vi "XY Graph Load Plot(s) Event.vi"(6 "Plot Format Information (dialog)":T1={"Number of Lines to Skip"=-1, "Column Header Line?"=FALSE, "Separator"="", "Abscissa Column?"=FALSE, "Abscissa Start"=nan, "Abscissa Step"=nan}, 7 "Max Number of Plot to Load (-1: All)":i32=-1, 8 "Error In":errorcluster, 9 "File Path":path, 10 "Used Dialog? (T)":bool=TRUE, 11 "XYGraph Ref":T2) -> (0 "Error Out":errorcluster, 1 "Message":string, 2 "File Path(s)":path[](array[path]), 3 "Loaded Plot Names":cluster{"Plot Names":string[]}[](array[cluster]), 4 "# Plots Added":i32[](array[numeric]), 5 "Graph Name":string)   [LabVIEW 2021, in "XY Graph Add-Ons.lvlib"]
uses:
  XY Graph Add-Ons.lvlib
  XY Graph Refnum.ctl
  XY Graph Plot Format Information.ctl
  Files/ASCII File Header Definition.ctl
  91129bd3-31c1-4cfb-ab33-95d83ad30e2f.vi
  0e8d2310-731b-4b54-9d07-3dcbb9077907.vi
  <vilib>/Utility/error.llb/Error Cluster From Error Code.vi
  XY Graph Get Plots Metadata.vi
  XY Graph Set Plots Metadata.vi
  <vilib>/ErrorRing/Error Ring.xnode
  Strings/Strings.lvlib
  Files/Files.lvlib
  Graphs.lvlib
  Error/Error.lvlib
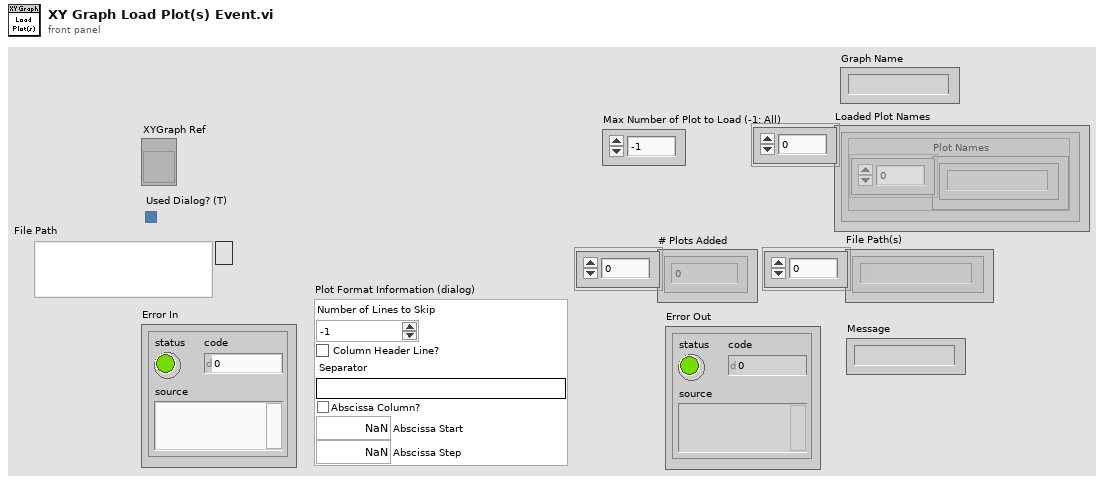
[diagram p1: front panel]
types:
  T1 = typedef "XY Graph Add-Ons.lvlib/XY Graph Plot Format Information.ctl" = cluster{"Number of Lines to Skip":i32, "Column Header Line?":bool, "Separator":string, "Abscissa Column?":bool, "Abscissa Start":dbl, "Abscissa Step":dbl}
  T2 = typedef "XY Graph Add-Ons.lvlib/XY Graph Refnum.ctl" = refnum<vi>
  T3 = typedef "Files.lvlib/ASCII File Header Definition.ctl" = cluster{"Number of Lines to Skip":i32, "Column Header Line?":bool}
  T4 = typedef "XY Graph Add-Ons.lvlib/XY Graph Plot Scale Labels.ctl" = cluster{"X Scale Label":string, "Y Scale Label":string}
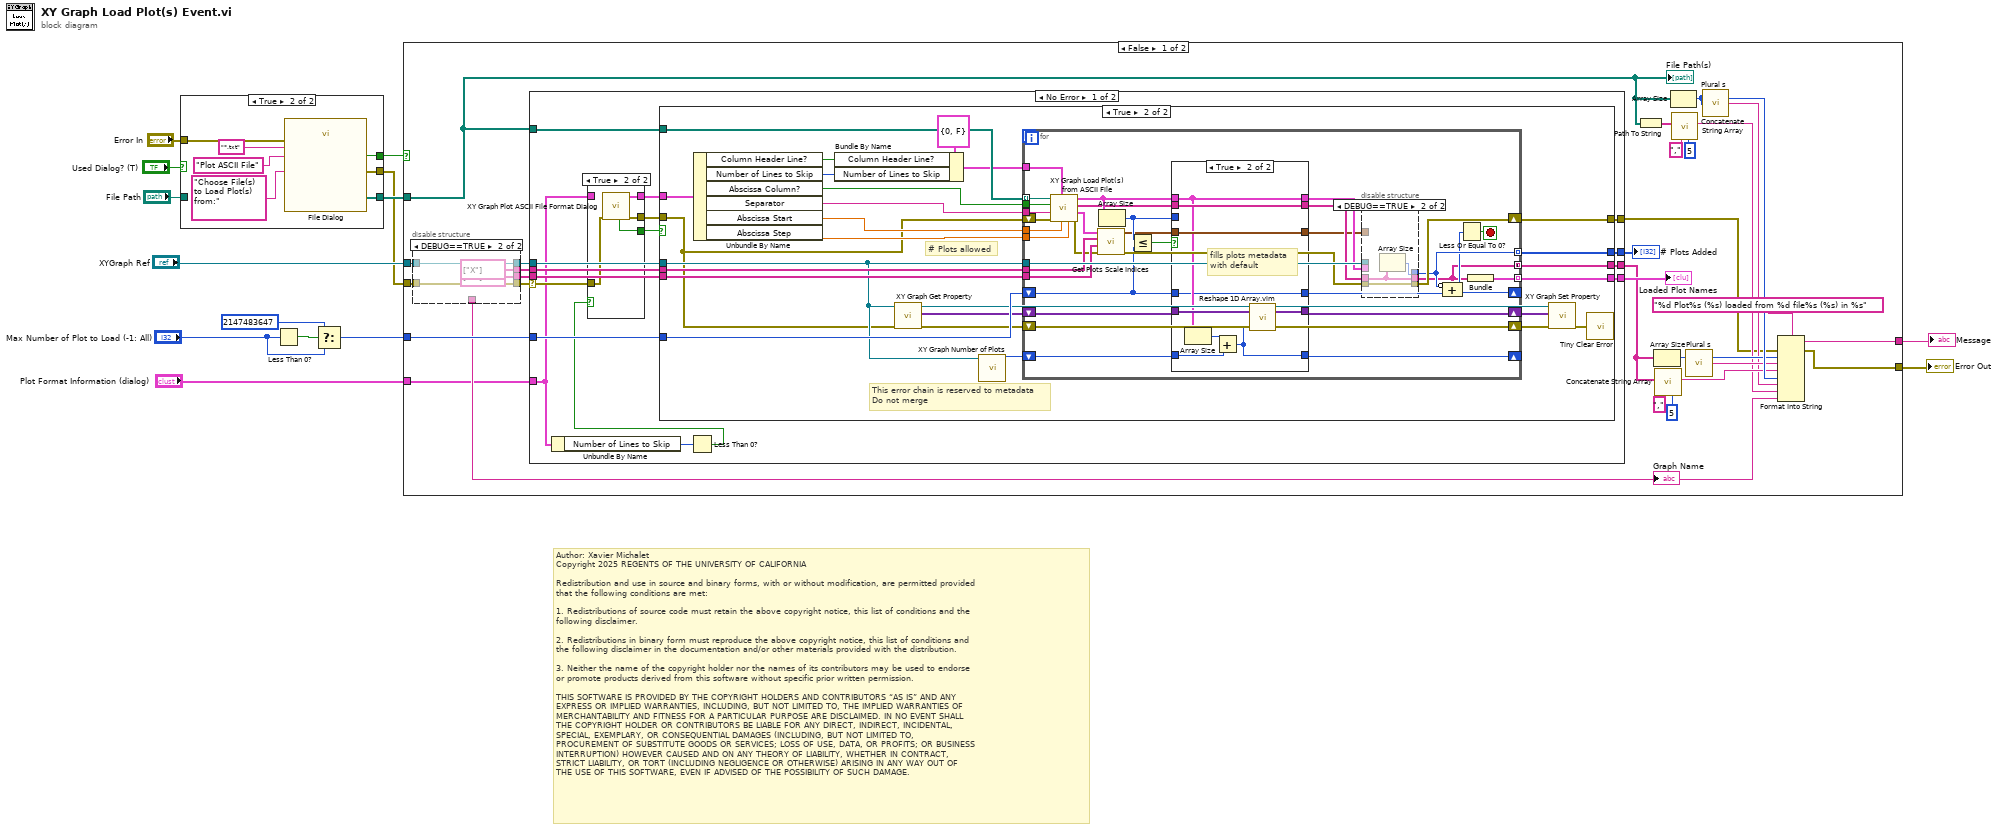
[diagram p0: block diagram]
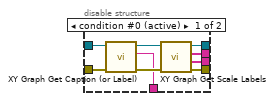
[diagram p2: hidden frame]
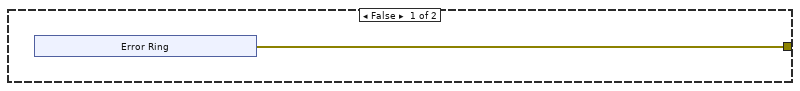
[diagram p4: hidden frame]
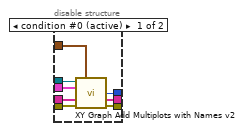
[diagram p5: hidden frame]
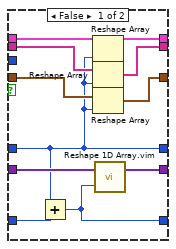
[diagram p6: hidden frame]
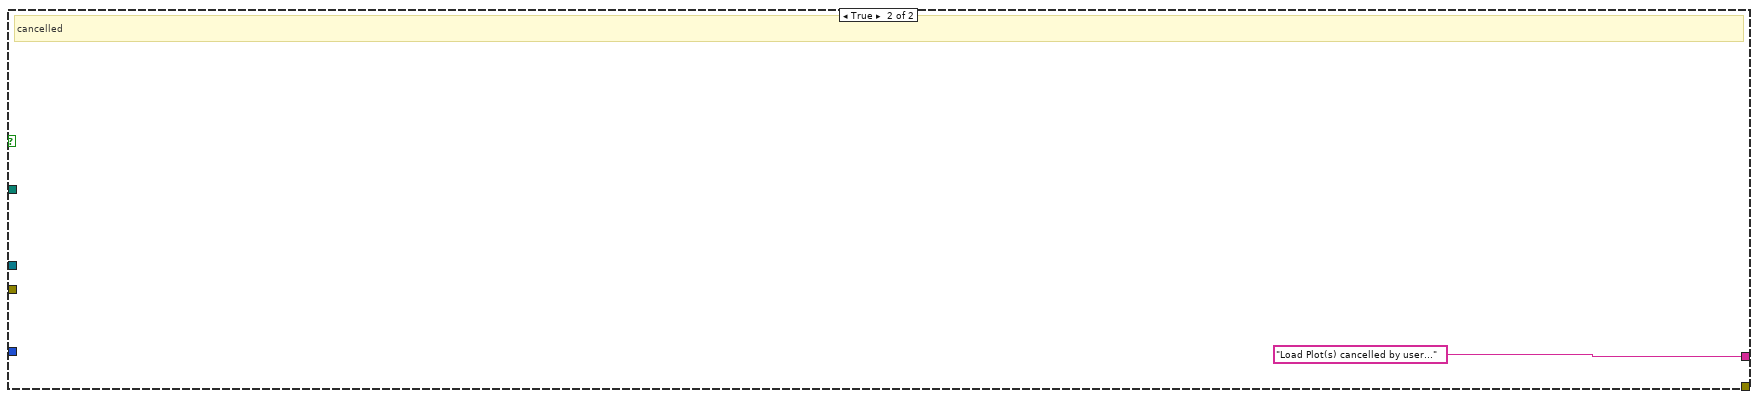
[diagram p8: hidden frame]
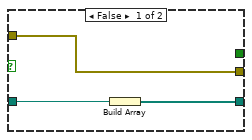
[diagram p9: hidden frame]
diagram:
  # "Author: Xavier Michalet\nCopyright 2025 REGENTS OF THE UNIVERSITY OF CALIFORNIA\n\nRedistribution and use in source and binary forms, with or without modification, are permitted provided\nthat the following conditions are met:\n\n1. Redistributions of source code must retain the above copyright notice, this list of conditions and the\nfollowing disclaimer.\n\n2. Redistributions in binary form must reproduce the above copyright notice, this list of conditions and\nthe following disclaimer in the documentation and/or other materials provided with the distribution.\n\n3. Neither the name of the copyright holder nor the names of its contributors may be used to endorse \nor promote products derived from this software without specific prior written permission.\n\nTHIS SOFTWARE IS PROVIDED BY THE COPYRIGHT HOLDERS AND CONTRIBUTORS “AS IS” AND ANY \nEXPRESS OR IMPLIED WARRANTIES, INCLUDING, BUT NOT LIMITED TO, THE IMPLIED WARRANTIES OF\nMERCHANTABILITY AND FITNESS FOR A PARTICULAR PURPOSE ARE DISCLAIMED. IN NO EVENT SHALL\nTHE COPYRIGHT HOLDER OR CONTRIBUTORS BE LIABLE FOR ANY DIRECT, INDIRECT, INCIDENTAL, \nSPECIAL, EXEMPLARY, OR CONSEQUENTIAL DAMAGES (INCLUDING, BUT NOT LIMITED TO, \nPROCUREMENT OF SUBSTITUTE GOODS OR SERVICES; LOSS OF USE, DATA, OR PROFITS; OR BUSINESS\nINTERRUPTION) HOWEVER CAUSED AND ON ANY THEORY OF LIABILITY, WHETHER IN CONTRACT, \nSTRICT LIABILITY, OR TORT (INCLUDING NEGLIGENCE OR OTHERWISE) ARISING IN ANY WAY OUT OF\nTHE USE OF THIS SOFTWARE, EVEN IF ADVISED OF THE POSSIBILITY OF SUCH DAMAGE."
  n1 = case shown="True" "Used Dialog? (T)" {
    tunnel: [w16 w21] -> w9
    tunnel: "Error In" -> [w15 w20]
    tunnel: [w15 w19] -> w5
    tunnel: "File Path" -> [w17 _]
    tunnel: [_ w18] -> w2
    frame False {
      n2 = Build Array(w17) -> (w16:path[])
    }
    frame True {
      n3 = call "File Dialog"("prompt"="Choose File(s) to Load Plot(s) from:", "error in"=w20, "pattern (all files)"="*.txt", "pattern label"="Plot ASCII File") -> ("selected paths"=w21:path[], "cancelled"=w18:bool, "error out"=w19:errorcluster)  [unwired: 8 in, 1 out]
    }
  }
  n4 = Less Than 0?(x="Max Number of Plot to Load (-1: All)") -> (x < 0?=w13:bool)
  n5 = Select(t=2147483647 ("Max Number of Plot to Load (-1: All)"), s=w13, f="Max Number of Plot to Load (-1: All)") -> (s? t:f=w10:i32)
  n6 = case shown="False" w2 {
    tunnel: "XYGraph Ref" -> [w52 _]
    tunnel: w10 -> [w46 _]
    tunnel: w9 -> [w38 _]
    tunnel: [w37 "Load Plot(s) cancelled by user..."] -> w8
    tunnel: [w28 _] -> w7
    tunnel: w5 -> [w27 _]
    tunnel: "Plot Format Information (dialog)" -> [w25 _]
    frame False {
      n7 = disable-structure shown="DEBUG==TRUE" {
        disable-tunnel: w52 -> [w61 w65]
        disable-tunnel: [w59 w65] -> w51
        disable-tunnel: [w58 string[] ["X"] ("X Scale Labels")] -> w50
        disable-tunnel: [w57 string[] ["Y"] ("Y Scale Labels")] -> w49
        disable-tunnel: [w55 _] -> w30
        disable-tunnel: w27 -> [w54 w64]
        disable-tunnel: [w53 w64] -> w26
        frame condition #0 (active) {
          n8 = call "XY Graph Get Caption (or Label).vi"("error in (no error)"=w54, "XY Graph in"=w61) -> ("error out"=w56:errorcluster, "Caption (or Label) Text"=w55:string, "XY Graph out"=w60:T2)  [unwired: 7 in]
          n9 = call "XY Graph Get Scale Labels.vi"("Error In"=w56, "XYGraph in"=w60) -> ("Error Out"=w53:errorcluster, "Y Scale Labels"=w57:string[], "X Scale Labels"=w58:string[], "XYGraph out"=w59:T2)  [unwired: 4 in, 2 out]
        }
        frame condition #1 {
        }
      }
      "Graph Name" <- w30
      n10 = case shown="No Error" w26 {
        selector: w26 -> [w81 w184]
        tunnel: w51 -> [w77 _]
        tunnel: w38 -> [w78 _]
        tunnel: [w76 _] -> w48
        tunnel: w50 -> [w75 _]
        tunnel: w49 -> [w74 _]
        tunnel: [w73 w184] -> w29
        tunnel: [w72 _] -> w47
        tunnel: w46 -> [w71 _]
        tunnel: [w70 _] -> w45
        tunnel: w25 -> [w68 _]
        frame No Error {
          n11 = Unbundle By Name(w68) -> ("Number of Lines to Skip"=w67:i32)
          n12 = Less Than 0?(x=w67) -> (x < 0?=w66:bool)
          n13 = case shown="True" w66 {
            tunnel: w81 -> [w82 w87]
            tunnel: [_ w86] -> w80
            tunnel: [w82 w85] -> w79
            tunnel: [w83 w84] -> w69
            tunnel: w68 -> [w83 _]
            frame False {
            }
            frame True {
              n14 = call "XY Graph Plot ASCII File Format Dialog.vi"("error in (no error)"=w87) -> ("error out"=w85:errorcluster, "Plot Format Information"=w84:T1, "OK"=w86:bool)  [unwired: 8 in]
            }
          }
          n15 = case shown="True" w80 {
            tunnel: w79 -> [_ w93]
            tunnel: w78 -> [_ w117]
            tunnel: w77 -> [_ w107]
            tunnel: [_ w118] -> w76
            tunnel: w75 -> [_ w114]
            tunnel: w74 -> [_ w113]
            tunnel: [w88 w112] -> w73
            tunnel: [_ w111] -> w72
            tunnel: w71 -> [_ w110]
            tunnel: [_ w109] -> w70
            tunnel: w69 -> [_ w101]
            frame False {
              n16 = xnode "Error Ring"() -> ("error out"=w88:errorcluster)
            }
            frame True {
              # "This error chain is reserved to metadata\nDo not merge"
              # "# Plots allowed"
              n17 = Unbundle By Name(w101) -> ("Column Header Line?"=w100:bool, "Number of Lines to Skip"=w99:i32, "Abscissa Column?"=w96:bool, "Separator"=w95:string, "Abscissa Start"=w98:dbl, "Abscissa Step"=w97:dbl)
              n18 = Bundle By Name(cluster=T3 {"Number of Lines to Skip"=0, "Column Header Line?"=FALSE} ("Header Definitions"), "Column Header Line?"=w100, "Number of Lines to Skip"=w99) -> (w115:T3)
              n19 = call-poly "XY Graph Get Property.vi"("Error In"=w93, "XYGraph Ref"=w107) -> ("Error Out"=w94:errorcluster, "Plot Metadata"=w108:variant[], "XYGraph Ref (dup)"=w103:T2)  [unwired: 6 in, 1 out]
              n20 = call "XY Graph Number of Plots.vi"("XYGraph in"=w107) -> ("# Plots"=w106:i32)  [unwired: 9 in, 1 out]
              n21 = for {
                tunnel: w107 -> [w152]
                tunnel: [w143] -> w118 mode=indexing
                tunnel: w117 -> [w151] mode=indexing
                tunnel: w95 -> [w123]
                tunnel: w115 -> [w149]
                tunnel: w114 -> [w148]
                tunnel: w113 -> [w147]
                shift-right: [w142] -> w112
                shift-left: w93 -> [w150]
                tunnel: [w136] -> w111 mode=indexing
                shift-right: [w135] -> _
                shift-left: w110 -> [w130]
                tunnel: [w129] -> w109 mode=concatenating
                shift-right: [w125] -> w105
                shift-left: w94 -> [w125]
                shift-right: [w126] -> w102
                shift-left: w108 -> [w128]
                shift-right: [w124] -> _
                shift-left: w106 -> [w127]
                tunnel: w97 -> [w120]
                tunnel: w98 -> [w122]
                tunnel: w96 -> [w119]
                stop <- w134 stop-if-true
                n22 = call "XY Graph Load Plot(s) from ASCII File.vi"("Default X step (1)"=w120, "Default X start (0)"=w122, "Header Definitions"=w149, "error in (no error)"=w150, "Delimiter (TAB)"=w123, "Abscissa Column? (T)"=w119, "File Path"=w151) -> ("error out"=w145:errorcluster, "Plot Scales Array"=w146:T4[], "Plot Name Array"=w138:string[], "Plot Array"=w139:cluster{"X Array":dbl[], "Y Array":dbl[]}[])  [unwired: 1 in]
                n23 = call "Get Plots Scale Indices.vi"("Error In"=w145, "Y Scale Labels"=w147, "X Scale Labels"=w148, "Plot Scales Array"=w146) -> ("Error Out"=w144:errorcluster, "Array of Scales (Default)"=w137:cluster{"X Scale":u32, "Y Scale":u32}[])  [unwired: 6 in]
                n24 = Array Size(array=w139) -> (size(s)=w140:i32)
                n25 = Less Or Equal?(x=w140, y=w130) -> (x <= y?=w141:bool)
                n26 = case shown="True" w141 {
                  tunnel: w140 -> [_ _]
                  tunnel: w139 -> [w174 w180]
                  tunnel: w138 -> [w170 w183]
                  tunnel: w137 -> [w172 w182]
                  tunnel: [w173 w180] -> w133
                  tunnel: [w169 w183] -> w132
                  tunnel: [w171 w182] -> w131
                  tunnel: w130 -> [w164 w175]
                  tunnel: w128 -> [w168 w181]
                  tunnel: w127 -> [w166 w178]
                  tunnel: [w167 w177] -> w126
                  tunnel: [w165 w176] -> w124
                  tunnel: [w164 w175] -> w121
                  frame False {
                    n27 = Add(x=w164, y=w166) -> (x+y=w165:i32)
                    n28 = Reshape Array(w174, w164) -> (w173:cluster{"X Array":dbl[], "Y Array":dbl[]}[])
                    n29 = Reshape Array(w170, w164) -> (w169:string[])
                    n30 = Reshape Array(w172, w164) -> (w171:cluster{"X Scale":u32, "Y Scale":u32}[])
                    n31 = call "Reshape 1D Array.vim"("dimension size"=w165, "1D Array"=w168) -> ("1D Array"=w167:variant[])  [unwired: 1 in]
                  }
                  frame True {
                    # "fills plots metadata\nwith default"
                    n32 = Array Size(array=w180) -> (size(s)=w179:i32)
                    n33 = Add(x=w179, y=w178) -> (x+y=w176:i32)
                    n34 = call "Reshape 1D Array.vim"("dimension size"=w176, "1D Array"=w181) -> ("1D Array"=w177:variant[])  [unwired: 1 in]
                  }
                }
                n35 = disable-structure shown="DEBUG==TRUE" {
                  disable-tunnel: w152 -> [w160 _]
                  disable-tunnel: w144 -> [w159 w163]
                  disable-tunnel: [w158 w163] -> w142
                  disable-tunnel: [w157 w161] -> w136
                  disable-tunnel: w133 -> [w156 _]
                  disable-tunnel: w132 -> [w155 w162]
                  disable-tunnel: w131 -> [w154 _]
                  disable-tunnel: [w153 w162] -> w129
                  frame condition #0 (active) {
                    n36 = call "XY Graph Add Multiplots with Names v2.vi"("XYGraph in"=w160, "Array of Scales (Default)"=w154, "Array of Plots"=w156, "Array of Plot Names (\"Plot\")"=w155, "error in (no error)"=w159) -> ("Number of Plots Added"=w157:i32, "Added Plot Names"=w153:string[], "error out"=w158:errorcluster)  [unwired: 6 in, 2 out]
                  }
                  frame condition #1 {
                    n37 = Array Size(array=w162) -> (size(s)=w161:i32)
                  }
                }
                n38 = Compound Arithmetic op=ADD(invert w136, w121) -> (w135:i32)
                n39 = Less Or Equal To 0?(x=w135) -> (x <= 0?=w134:bool)
                n40 = Bundle("Added Plot Names"=w129) -> (w143:cluster{"Added Plot Names":string[]})  [unwired: 1 in]
              }
              n41 = call-poly "XY Graph Set Property.vi"("error in (no error)"=w105, "Plots Metadata"=w102, "XY Graph Refnum"=w103) -> ("error out"=w104:errorcluster)  [unwired: 7 in, 1 out]
              n42 = call "Tiny Clear Error.vi"("Error In"=w104) -> ()  [unwired: 8 in, 1 out]
            }
          }
        }
        frame Error {
        }
      }
      "Loaded Plot Names" <- w48
      "# Plots Added" <- w47
      n43 = Path To String(path=w38) -> (string=w39:string[])
      n44 = Array Size(array=w45) -> (size(s)=w35:i32)
      n45 = call "Concatenate String Array.vi"("Max Number of Elements (None: -1)"=5 ("Max Number of Elements (None: 1)"), "Separator (TAB)"=",", "String Array"=w45) -> ("Formatted String"=w33:string)  [unwired: 8 in]
      n46 = Array Size(array=w38) -> (size(s)=w36:i32)
      n47 = call "Concatenate String Array.vi"("Max Number of Elements (None: -1)"=5 ("Max Number of Elements (None: 1)"), "Separator (TAB)"=",", "String Array"=w39) -> ("Formatted String"=w32:string)  [unwired: 8 in]
      n48 = call "Plural s.vi"("# Elements"=w35) -> ("Plural s"=w34:string)
      n49 = call "Plural s.vi"("# Elements"=w36) -> ("Plural s"=w31:string)
      n50 = Format Into String(format string="%d Plot%s (%s) loaded from %d file%s (%s) in %s", error in=w29, w35, w34, w33, w36, w31, w32, w30) -> (resulting string=w37:string, error out=w28:errorcluster)  [unwired: 1 in]
      "File Path(s)" <- w38
    }
    frame True {
      # "cancelled"
    }
  }
  "Error Out" <- w7
  "Message" <- w8
